vi "FoundInstruments.vi"(8 "error in (no error)":errorcluster, 10 "FoundInstruments":T2(array[cluster]), 11 "SpectroscopyUI in":refnum<class "SpectroscopyUI.lvclass">) -> (0 "error out":errorcluster, 3 "SpectroscopyUI out":refnum<class "SpectroscopyUI.lvclass">)   [LabVIEW 2023, in "SpectroscopyUI.lvlib" / "SpectroscopyUI.lvclass"]
uses:
  SpectroscopyUI.lvclass
  SpectroscopyUI.lvclass/SpectroscopyUI.ctl
  InterferometryUI/InterferometryUI/instrumentType.ctl
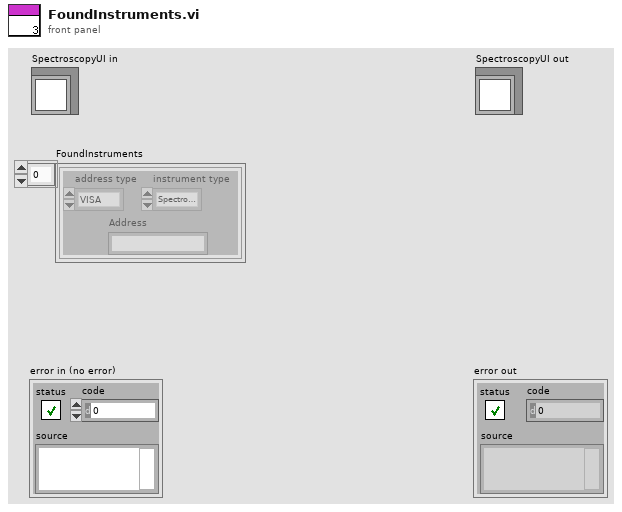
[diagram p1: front panel]
types:
  T1 = typedef "instrumentType.ctl" = enum16{"Spectrometer", "Camera", "Stepper"}
  T2 = cluster{"address type":enum16{"VISA", "Index"}, "Address":string, "instrument type":T1}[]
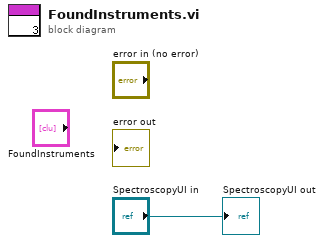
[diagram p0: block diagram]
diagram:
  "SpectroscopyUI out" <- "SpectroscopyUI in"
